vi "Configure Module.vi"(8 "error in (no error)":errorcluster, 10 "IOV ref in":refnum<k21>, 11 "Module Template in":refnum<class "9205.lvclass">) -> (0 "error out":errorcluster, 2 "IOV ref out":refnum<k21>, 3 "Module Template out":refnum<class "9205.lvclass">)   [LabVIEW 2019, in "Modules.lvlib" / "9205.lvclass"]
uses:
  9205.lvclass
  C:/Users/nitest/Desktop/Git 2019/niveristand-scan-engine-module-libraries/Source/RSI Module/RSI Module.lvclass
  9205.lvclass/9205.ctl
  <resource>/objmgr/cRIO.rc
  RSI Module/RSI Module.lvclass
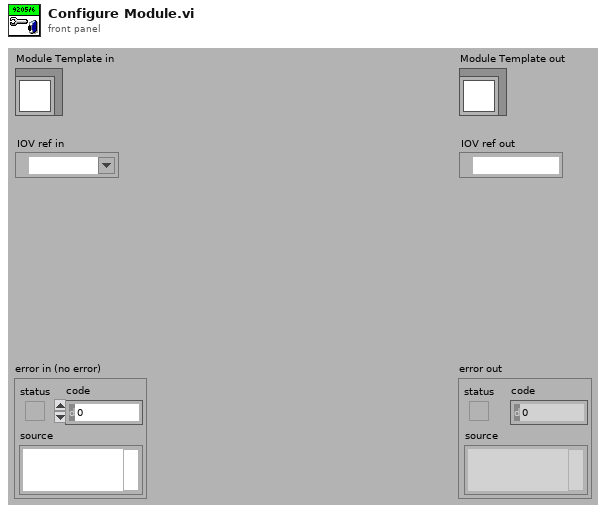
[diagram p1: front panel]
types:
  T1 = typedef "Modules.lvlib/9205.lvclass/Channel Settings.ctl" = cluster{"Range":T2, "Terminal mode":T3}[]
  T2 = typedef "Modules.lvlib/9205.lvclass/Range.ctl" = u32
  T3 = typedef "Modules.lvlib/9205.lvclass/Terminal mode.ctl" = u32
  T4 = typedef "Modules.lvlib/RSI Module.lvclass/Module Models.ctl" = enum16{"Empty", "NI 9201", "NI 9203", "NI 9205", "NI 9206", "NI 9207", "NI 9208", "NI 9209", "NI 9210", "NI 9211", "NI 9212", "NI 9213", "NI 9214", "NI 9215", "NI 9216", "NI 9217", "NI 9219", "NI 9220", "NI 9221", "NI 9222", "NI 9223", "NI 9224", "NI 9225", "NI 9226", "NI 9227", "NI 9228", "NI 9229", "NI 9233", "NI 9234", "NI 9235", "NI 9236", "NI 9237", "NI 9239", "NI 9242", "NI 9244", "NI 9253", "NI 9263", "NI 9264", "NI 9265", "NI 9266", "NI 9269", "NI 9344", "NI 9350", "NI 9375", "NI 9401", "NI 9402", "NI 9403", "NI 9411", "NI 9421", "NI 9422", "NI 9423", "NI 9425", "NI 9426", "NI 9435", "NI 9436", "NI 9437", "NI 9472", "NI 9474", "NI 9475", "NI 9476", "NI 9477", "NI 9478", "NI 9481", "NI 9482", "NI 9485"}
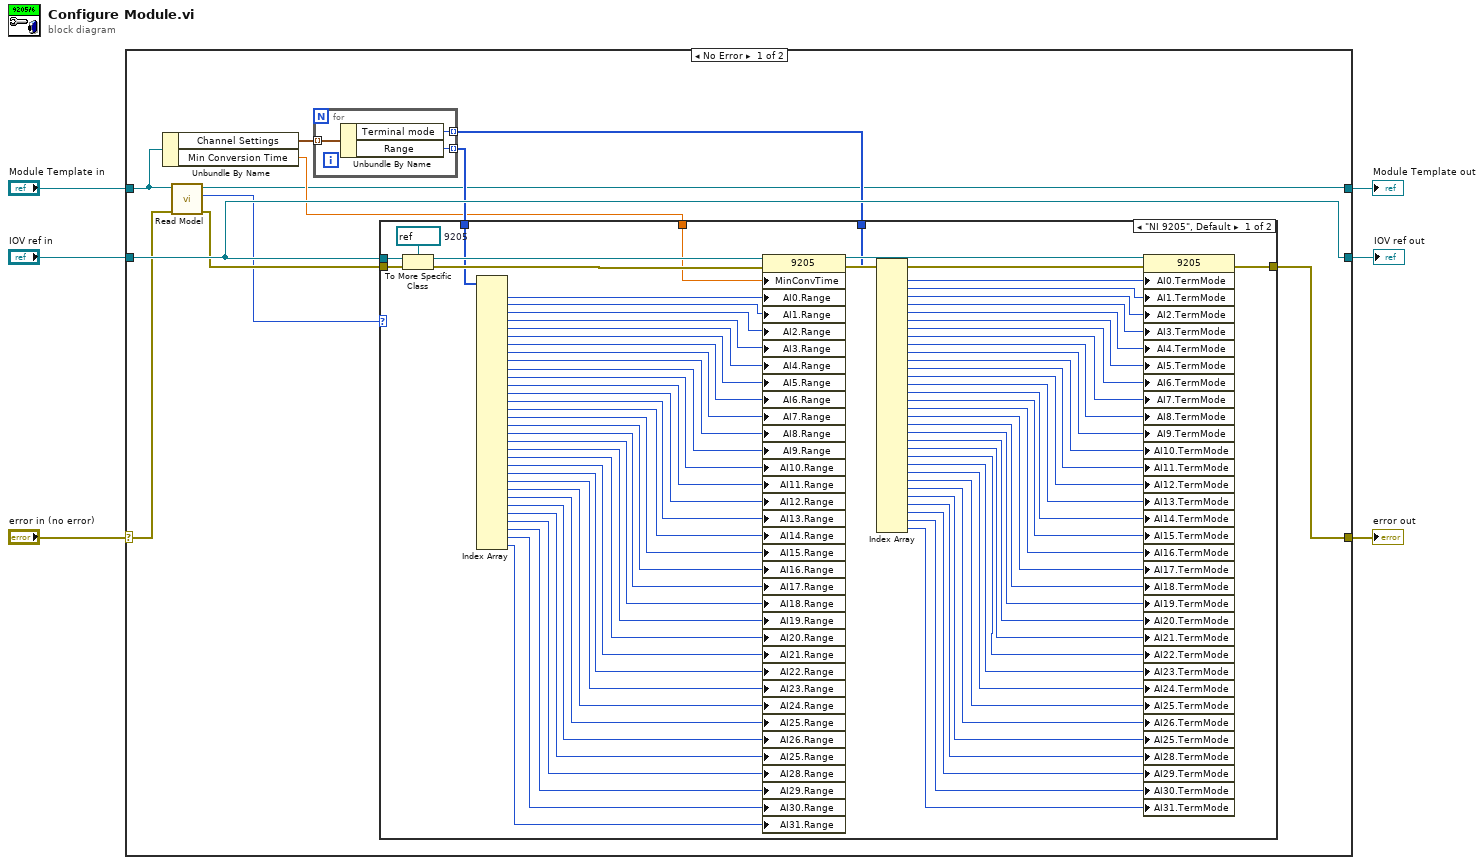
[diagram p0: block diagram]
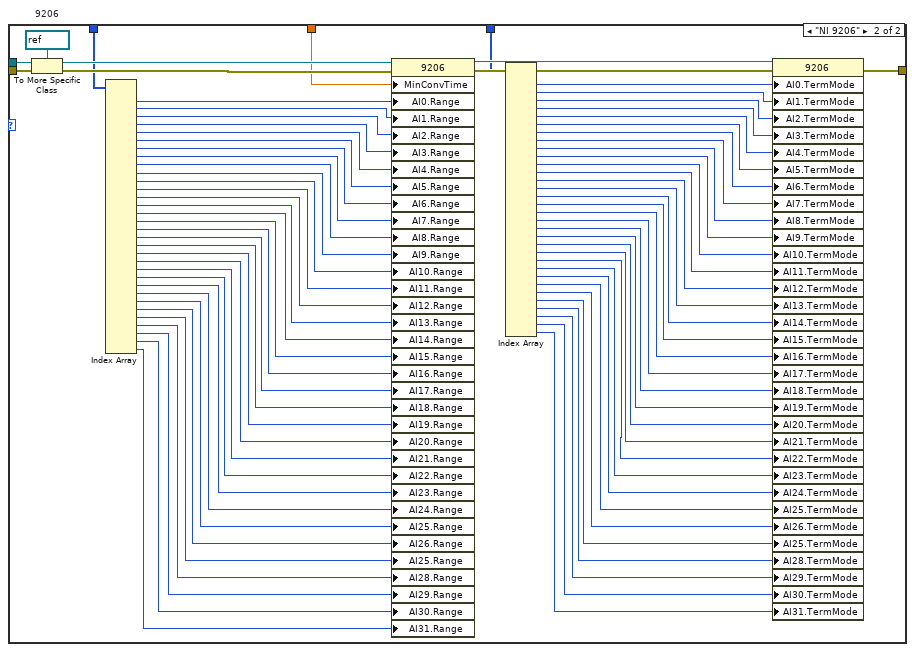
[diagram p2: hidden frame]
diagram:
  n1 = case shown="No Error" "error in (no error)" {
    selector: "error in (no error)" -> [w9 w173]
    tunnel: [w15 w173] -> w5
    tunnel: [w10 w172] -> w3
    tunnel: "Module Template in" -> [w11 w172]
    tunnel: "IOV ref in" -> [w17 w171]
    tunnel: [w17 w171] -> w1
    frame No Error {
      n2 = Unbundle By Name(w11) -> ("Channel Settings"=w16:T1, "Min Conversion Time"=w12:dbl)
      n3 = call "Read Model.vi"("error in (no error)"=w9, "RSI Module in"=w11) -> ("error out"=w8:errorcluster, "Model"=w7:T4, "RSI Module out"=w10:refnum<class "9205.lvclass">)  [unwired: 7 in]
      n4 = for {
        tunnel: w16 -> [w170] mode=indexing
        tunnel: [w169] -> w13 mode=indexing
        tunnel: [w168] -> w14 mode=indexing
        n5 = Unbundle By Name(w170) -> ("Terminal mode"=w169:T3, "Range"=w168:T2)
      }
      n6 = case shown="\"NI 9205\", Default" w7 {
        tunnel: w8 -> [w92 w167]
        tunnel: w17 -> [w88 w163]
        tunnel: [w85 w160] -> w15
        tunnel: w14 -> [w84 w159]
        tunnel: w13 -> [w52 w127]
        tunnel: w12 -> [w50 w125]
        frame "NI 9205", Default {
          w91 = refnum<k21> refnum  # 9205
          n7 = To More Specific Class(target class=w91, reference=w88, error in=w92) -> (specific class reference=w90:refnum<k21>, error out=w89:errorcluster)
          n8 = Index Array(array=w84) -> (element #1=w51:T2, element #2=w83:T2, element #3=w82:T2, element #4=w81:T2, element #5=w80:T2, element #6=w79:T2, element #7=w78:T2, element #8=w77:T2, element #9=w76:T2, element #10=w75:T2, element #11=w74:T2, element #12=w73:T2, element #13=w72:T2, element #14=w71:T2, element #15=w70:T2, element #16=w69:T2, element #17=w68:T2, element #18=w67:T2, element #19=w66:T2, element #20=w65:T2, element #21=w64:T2, element #22=w63:T2, element #23=w62:T2, element #24=w61:T2, element #25=w60:T2, element #26=w59:T2, element #27=w58:T2, element #28=w57:T2, element #29=w56:T2, element #30=w55:T2, element #31=w54:T2, element #32=w53:T2)  [unwired: 32 in]
          n9 = property class="9205"(reference=w90, error in=w89, "MinConvTime"=w50, "AI0.Range"=w51, "AI1.Range"=w83, "AI2.Range"=w82, "AI3.Range"=w81, "AI4.Range"=w80, "AI5.Range"=w79, "AI6.Range"=w78, "AI7.Range"=w77, "AI8.Range"=w76, "AI9.Range"=w75, "AI10.Range"=w74, "AI11.Range"=w73, "AI12.Range"=w72, "AI13.Range"=w71, "AI14.Range"=w70, "AI15.Range"=w69, "AI16.Range"=w68, "AI17.Range"=w67, "AI18.Range"=w66, "AI19.Range"=w65, "AI20.Range"=w64, "AI21.Range"=w63, "AI22.Range"=w62, "AI23.Range"=w61, "AI24.Range"=w60, "AI25.Range"=w59, "AI26.Range"=w58, "AI25.Range"=w57, "AI28.Range"=w56, "AI29.Range"=w55, "AI30.Range"=w54, "AI31.Range"=w53) -> (reference out=w87:refnum<k21>, error out=w86:errorcluster)
          n10 = Index Array(array=w52) -> (element #1=w49:T3, element #2=w48:T3, element #3=w47:T3, element #4=w46:T3, element #5=w45:T3, element #6=w44:T3, element #7=w43:T3, element #8=w42:T3, element #9=w41:T3, element #10=w40:T3, element #11=w39:T3, element #12=w38:T3, element #13=w37:T3, element #14=w36:T3, element #15=w35:T3, element #16=w34:T3, element #17=w33:T3, element #18=w32:T3, element #19=w31:T3, element #20=w30:T3, element #21=w29:T3, element #22=w28:T3, element #23=w27:T3, element #24=w26:T3, element #25=w25:T3, element #26=w24:T3, element #27=w23:T3, element #28=w22:T3, element #29=w21:T3, element #30=w20:T3, element #31=w19:T3, element #32=w18:T3)  [unwired: 32 in]
          n11 = property class="9205"(reference=w87, error in=w86, "AI0.TermMode"=w49, "AI1.TermMode"=w48, "AI2.TermMode"=w47, "AI3.TermMode"=w46, "AI4.TermMode"=w45, "AI5.TermMode"=w44, "AI6.TermMode"=w43, "AI7.TermMode"=w42, "AI8.TermMode"=w41, "AI9.TermMode"=w40, "AI10.TermMode"=w39, "AI11.TermMode"=w38, "AI12.TermMode"=w37, "AI13.TermMode"=w36, "AI14.TermMode"=w35, "AI15.TermMode"=w34, "AI16.TermMode"=w33, "AI17.TermMode"=w32, "AI18.TermMode"=w31, "AI19.TermMode"=w30, "AI20.TermMode"=w29, "AI21.TermMode"=w28, "AI22.TermMode"=w27, "AI23.TermMode"=w26, "AI24.TermMode"=w25, "AI25.TermMode"=w24, "AI26.TermMode"=w23, "AI25.TermMode"=w22, "AI28.TermMode"=w21, "AI29.TermMode"=w20, "AI30.TermMode"=w19, "AI31.TermMode"=w18) -> (error out=w85:errorcluster)  [unwired: 1 out]
        }
        frame "NI 9206" {
          w166 = refnum<k21> refnum  # 9206
          n12 = To More Specific Class(target class=w166, reference=w163, error in=w167) -> (specific class reference=w165:refnum<k21>, error out=w164:errorcluster)
          n13 = Index Array(array=w159) -> (element #1=w126:T2, element #2=w158:T2, element #3=w157:T2, element #4=w156:T2, element #5=w155:T2, element #6=w154:T2, element #7=w153:T2, element #8=w152:T2, element #9=w151:T2, element #10=w150:T2, element #11=w149:T2, element #12=w148:T2, element #13=w147:T2, element #14=w146:T2, element #15=w145:T2, element #16=w144:T2, element #17=w143:T2, element #18=w142:T2, element #19=w141:T2, element #20=w140:T2, element #21=w139:T2, element #22=w138:T2, element #23=w137:T2, element #24=w136:T2, element #25=w135:T2, element #26=w134:T2, element #27=w133:T2, element #28=w132:T2, element #29=w131:T2, element #30=w130:T2, element #31=w129:T2, element #32=w128:T2)  [unwired: 32 in]
          n14 = property class="9206"(reference=w165, error in=w164, "MinConvTime"=w125, "AI0.Range"=w126, "AI1.Range"=w158, "AI2.Range"=w157, "AI3.Range"=w156, "AI4.Range"=w155, "AI5.Range"=w154, "AI6.Range"=w153, "AI7.Range"=w152, "AI8.Range"=w151, "AI9.Range"=w150, "AI10.Range"=w149, "AI11.Range"=w148, "AI12.Range"=w147, "AI13.Range"=w146, "AI14.Range"=w145, "AI15.Range"=w144, "AI16.Range"=w143, "AI17.Range"=w142, "AI18.Range"=w141, "AI19.Range"=w140, "AI20.Range"=w139, "AI21.Range"=w138, "AI22.Range"=w137, "AI23.Range"=w136, "AI24.Range"=w135, "AI25.Range"=w134, "AI26.Range"=w133, "AI25.Range"=w132, "AI28.Range"=w131, "AI29.Range"=w130, "AI30.Range"=w129, "AI31.Range"=w128) -> (reference out=w162:refnum<k21>, error out=w161:errorcluster)
          n15 = Index Array(array=w127) -> (element #1=w124:T3, element #2=w123:T3, element #3=w122:T3, element #4=w121:T3, element #5=w120:T3, element #6=w119:T3, element #7=w118:T3, element #8=w117:T3, element #9=w116:T3, element #10=w115:T3, element #11=w114:T3, element #12=w113:T3, element #13=w112:T3, element #14=w111:T3, element #15=w110:T3, element #16=w109:T3, element #17=w108:T3, element #18=w107:T3, element #19=w106:T3, element #20=w105:T3, element #21=w104:T3, element #22=w103:T3, element #23=w102:T3, element #24=w101:T3, element #25=w100:T3, element #26=w99:T3, element #27=w98:T3, element #28=w97:T3, element #29=w96:T3, element #30=w95:T3, element #31=w94:T3, element #32=w93:T3)  [unwired: 32 in]
          n16 = property class="9206"(reference=w162, error in=w161, "AI0.TermMode"=w124, "AI1.TermMode"=w123, "AI2.TermMode"=w122, "AI3.TermMode"=w121, "AI4.TermMode"=w120, "AI5.TermMode"=w119, "AI6.TermMode"=w118, "AI7.TermMode"=w117, "AI8.TermMode"=w116, "AI9.TermMode"=w115, "AI10.TermMode"=w114, "AI11.TermMode"=w113, "AI12.TermMode"=w112, "AI13.TermMode"=w111, "AI14.TermMode"=w110, "AI15.TermMode"=w109, "AI16.TermMode"=w108, "AI17.TermMode"=w107, "AI18.TermMode"=w106, "AI19.TermMode"=w105, "AI20.TermMode"=w104, "AI21.TermMode"=w103, "AI22.TermMode"=w102, "AI23.TermMode"=w101, "AI24.TermMode"=w100, "AI25.TermMode"=w99, "AI26.TermMode"=w98, "AI25.TermMode"=w97, "AI28.TermMode"=w96, "AI29.TermMode"=w95, "AI30.TermMode"=w94, "AI31.TermMode"=w93) -> (error out=w160:errorcluster)  [unwired: 1 out]
        }
      }
    }
    frame Error {
    }
  }
  "error out" <- w5
  "Module Template out" <- w3
  "IOV ref out" <- w1
